vi "Create - I16 Array.vi"(6 "timestamp":timestamp, 7 "fields":T1, 8 "error in (no error)":errorcluster, 10 "value":i16[](array[numeric])) -> (0 "error out":errorcluster, 3 "NT Scalar (Numeric) out":refnum<class "NT Scalar (Numeric).lvclass">)   [LabVIEW 2020, in "PV Access.lvlib" / "PV Data.lvlib" / "NT Scalar (Numeric).lvclass"]
uses:
  NT Scalar (Numeric).lvclass
  NT Scalar (Numeric).lvclass/NT Scalar (Numeric).ctl
  8ca984eb-dd67-4c23-9022-91f86214c627.vi
  Value Fields.ctl
  PV Data.lvlib
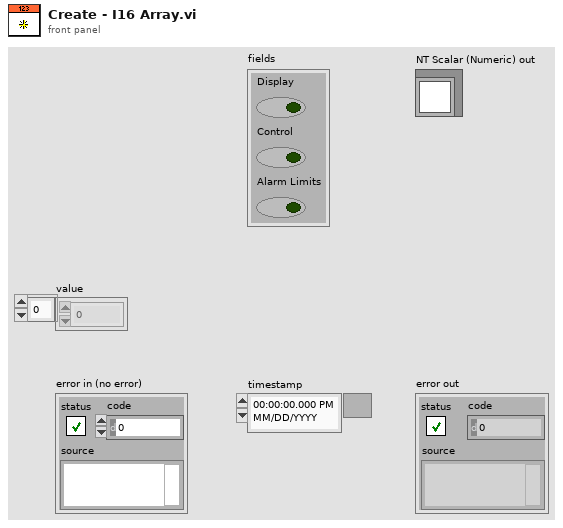
[diagram p1: front panel]
types:
  T1 = typedef "PV Access.lvlib/PV Data.lvlib/Value Fields.ctl" = cluster{"Display":bool, "Control":bool, "Alarm Limits":bool}
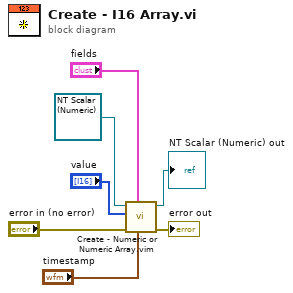
[diagram p0: block diagram]
diagram:
  n1 = call "Create - Numeric or Numeric Array.vim"("time stamp"="timestamp", "value fields"="fields", "error in (no error)"="error in (no error)", "value"="value", "NT Scalar (Numeric) in"=refnum<class "NT Scalar (Numeric).lvclass"> refnum) -> ("error out"=→"error out":errorcluster, "NT Scalar (Numeric) out"=→"NT Scalar (Numeric) out":refnum<class "NT Scalar (Numeric).lvclass">)  [unwired: 5 in]
